vi "sin_data_plotter.vi"(6 "subtract-mean":bool=TRUE, 7 "freq_adjusted?":dbl, 8 "error in (no error)":errorcluster, 10 "sin-data-out":dbl[][](array[numeric]), 11 "time-series figures (in)":T1) -> (0 "error out":errorcluster, 3 "time-series figures (out)":T1)   [LabVIEW 2017]
uses:
  labview/sysID/controls/time_series_figures.ctl
panel:
  out "t_final":dbl format="%#_13g"
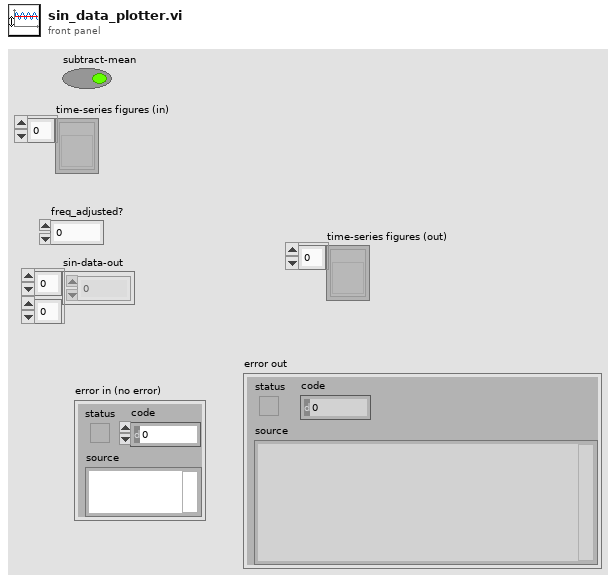
[diagram p1: front panel]
types:
  T1 = typedef "time_series_figures.ctl" = refnum<vi>[]
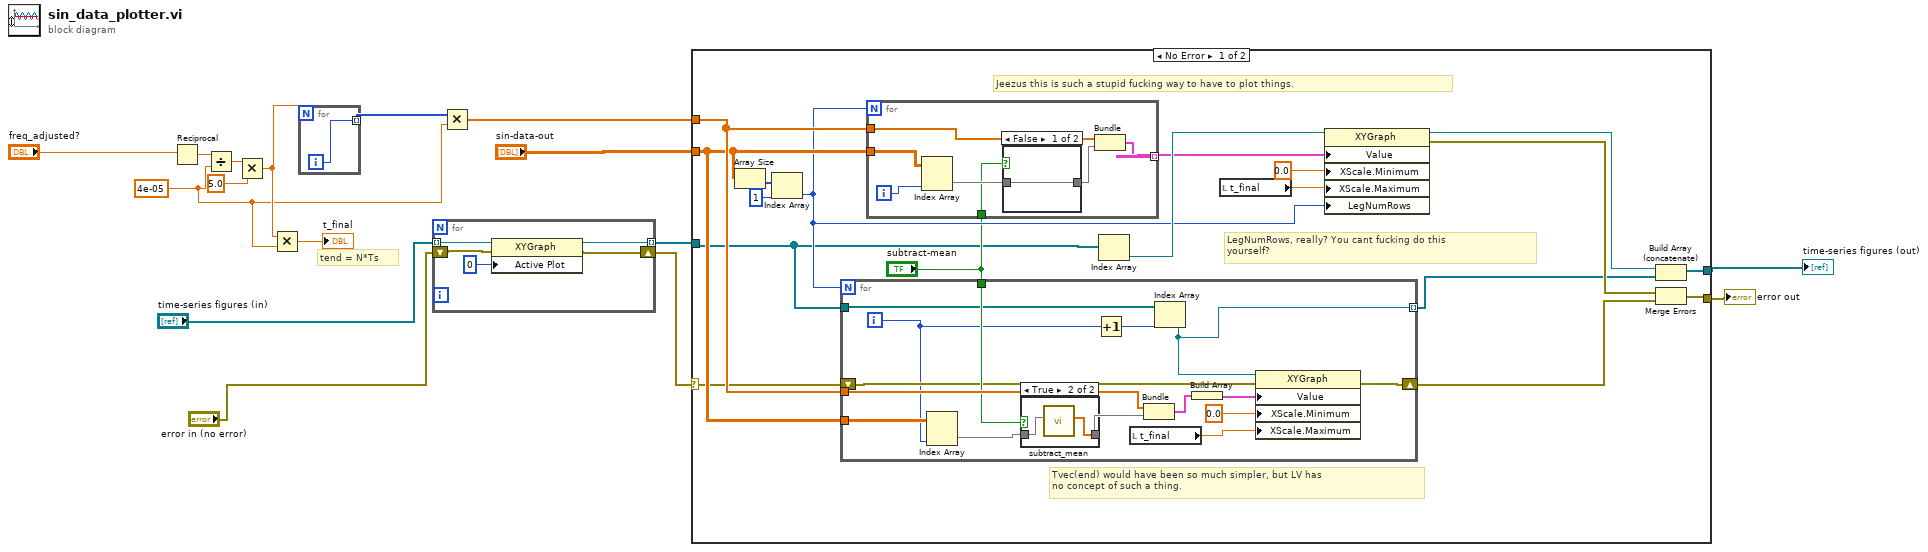
[diagram p0: block diagram]
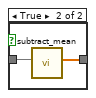
[diagram p3: hidden frame]
diagram:
  w7 = 4e-05
  # "tend = N*Ts"
  n1 = Reciprocal(x="freq_adjusted?") -> (1/x=w14:dbl)
  n2 = Divide(x=w14, y=w7) -> (x/y=w13:dbl)
  n3 = Multiply(x=w13, y=5.0) -> (x*y=w8:dbl)
  n4 = Multiply(x=w8, y=w7) -> (x*y=→"t_final":dbl)
  n5 = for {
    N: w8 -> [_]
    tunnel: [w17] -> w11 mode=indexing
    i -> [w17]
  }
  n6 = for {
    tunnel: [w22] -> w5 mode=indexing
    tunnel: "time-series figures (in)" -> [w20] mode=indexing
    shift-right: [w18] -> w1
    shift-left: "error in (no error)" -> [w19]
    n7 = property class="XYGraph"(reference=w20, error in=w19, "Active Plot"=u32 0) -> (reference out=w22:refnum<vi>, error out=w18:errorcluster)
  }
  n8 = Multiply(x=w11, y=w7) -> (x*y=w9:dbl[])
  n9 = case shown="No Error" w1 {
    selector: w1 -> [w25 w70]
    tunnel: [w37 w69] -> w3
    tunnel: [w33 w70] -> w16
    tunnel: "sin-data-out" -> [w30 _]
    tunnel: w9 -> [w39 _]
    tunnel: w5 -> [w24 w69]
    frame No Error {
      # "Tvec(end) would have been so much simpler, but LV has\nno concept of such a thing."
      # "LegNumRows, really? You cant fucking do this\nyourself?"
      # "Jeezus this is such a stupid fucking way to have to plot things."
      n10 = Array Size(array=w30) -> (size(s)=w29:i32[])
      n11 = Index Array(array=w29, index=1) -> (element=w27:i32)
      n12 = for {
        N: w27 -> [_]
        tunnel: w39 -> [w55]
        tunnel: w30 -> [w54]
        tunnel: "subtract-mean" -> [w46]
        shift-right: [w44] -> w38
        shift-left: w25 -> [w45]
        tunnel: w24 -> [w42]
        tunnel: [w41] -> w23 mode=indexing
        i -> [w43]
        n13 = Index Array(array=w54, index (col)=w43) -> (element=w48:dbl[])  [unwired: 1 in]
        n14 = case shown="True" w46 {
          tunnel: [w56 w58] -> w47
          tunnel: w48 -> [w56 w57]
          frame False {
          }
          frame True {
            n15 = call "subtract_mean.vi"("X"=w57) -> ("x-y"=w58:dbl[])  [unwired: 10 in]
          }
        }
        n16 = Increment(x=w43) -> (x+1=w49:i32)
        n17 = local read "t_final"() -> (w50:dbl)
        n18 = Bundle(w55, "x-y"=w47) -> (w52:cluster{dbl[], "x-y":dbl[]})  [unwired: 1 in]
        n19 = Index Array(array=w42, index=w49) -> (element=w41:refnum<vi>)
        n20 = Build Array(w52) -> (w53:cluster{dbl[], "x-y":dbl[]}[])
        n21 = property class="XYGraph"(reference=w41, error in=w45, "Value"=w53, "XScale.Minimum"=0.0 ("X Scale.Range:Minimum"), "XScale.Maximum"=w50) -> (error out=w44:errorcluster)  [unwired: 1 out]
      }
      n22 = for {
        N: w27 -> [_]
        tunnel: w39 -> [w65]
        tunnel: w30 -> [w64]
        tunnel: [w63] -> w34 mode=indexing
        tunnel: "subtract-mean" -> [w59]
        i -> [w62]
        n23 = Index Array(array=w64, index (col)=w62) -> (element=w60:dbl[])  [unwired: 1 in]
        n24 = case shown="False" w59 {
          tunnel: [w66 w68] -> w61
          tunnel: w60 -> [w66 w67]
          frame False {
          }
          frame True {
            n25 = call "subtract_mean.vi"("X"=w67) -> ("x-y"=w68:dbl[])  [unwired: 10 in]
          }
        }
        n26 = Bundle(w65, "x-y"=w61) -> (w63:cluster{dbl[], "x-y":dbl[]})  [unwired: 1 in]
      }
      n27 = Index Array(array=w24) -> (element=w40:refnum<vi>)  [unwired: 1 in]
      n28 = local read "t_final"() -> (w36:dbl)
      n29 = property class="XYGraph"(reference=w40, "Value"=w34, "XScale.Minimum"=0.0 ("X Scale.Range:Minimum"), "XScale.Maximum"=w36, "LegNumRows"=w27) -> (reference out=w32:refnum<vi>, error out=w31:errorcluster)  [unwired: 1 in]
      n30 = Build Array (concatenate)(w32, w23) -> (w37:refnum<vi>[])
      n31 = Merge Errors(w31, w38) -> (w33:errorcluster)
    }
    frame Error {
    }
  }
  "error out" <- w16
  "time-series figures (out)" <- w3
